vi "Cockpit_Demo.vi"() -> ()   [LabVIEW 2012]
uses:
  Sub_VIs/Instruments/SlipIndicator.ctl
  Sub_VIs/IMU_Functions/IMU_Data_Cluster.ctl
panel:
  in  "GPS/Baro_Vario":bool
  in  "GPS/Mag":bool
  in  "GPS/Baro_Alt":bool
  in  "ScaleUnit(F=m; T=feet)":bool
  out "AltitudeIndicator":picture
  out "VerticalSpeedIndicator":picture
  out "TurnBankPlaneIndicator":picture caption="Neue Grafik"
  in  "ScaleUnit(F=km/h; T=knots)":bool
  out "SpeedIndicator":picture
  out "TurnBankStdRate":bool
  out "AltitudeDigital":dbl
  out "VerticalSpeedDigital":dbl format="%.1f"
  out "HeadingDigital":dbl format="%.1f"
  out "Compass":picture
  in  "MultiWii Data Cluster":T1 {"Altitude abs [m]" format="%.2f"; "Baro T [°C]" format="%.1f"; "Baro P [mbara]" format="%.1f"; "GPS_coord[LON]" format="%#_9f"; "GPS_coord[LAT]" format="%#_9f"; "Altitude [m]" format="%.2f"}
  in  "SlipIndicator":dbl(knob) scale=-10.0..10.0
  out "GPS Data Valid?":bool
  out "GPS Sensor OK":bool
  out "UTC":string
  out "Local":string
  in  "Difference Local/UTC [h]":i32=1
  in  "Reset":bool
  in  "EXIT":bool
  in  "AH-Roll":dbl(knob) scale=-180.0..180.0
  in  "AH-Pitch":dbl(knob) scale=-90.0..90.0
  in  "Altitude":dbl(knob) scale=0.0..15000.0
  in  "Vert.Speed":dbl(knob) scale=-20.0..20.0
  in  "Kompass":dbl(knob) scale=0.0..360.0
  in  "Speed":dbl(knob) scale=0.0..200.0
  out "SlipIndicator":T2 scale=-10.0..10.0
  out "ArtificialHorizon":picture
  # "D - CF2811"
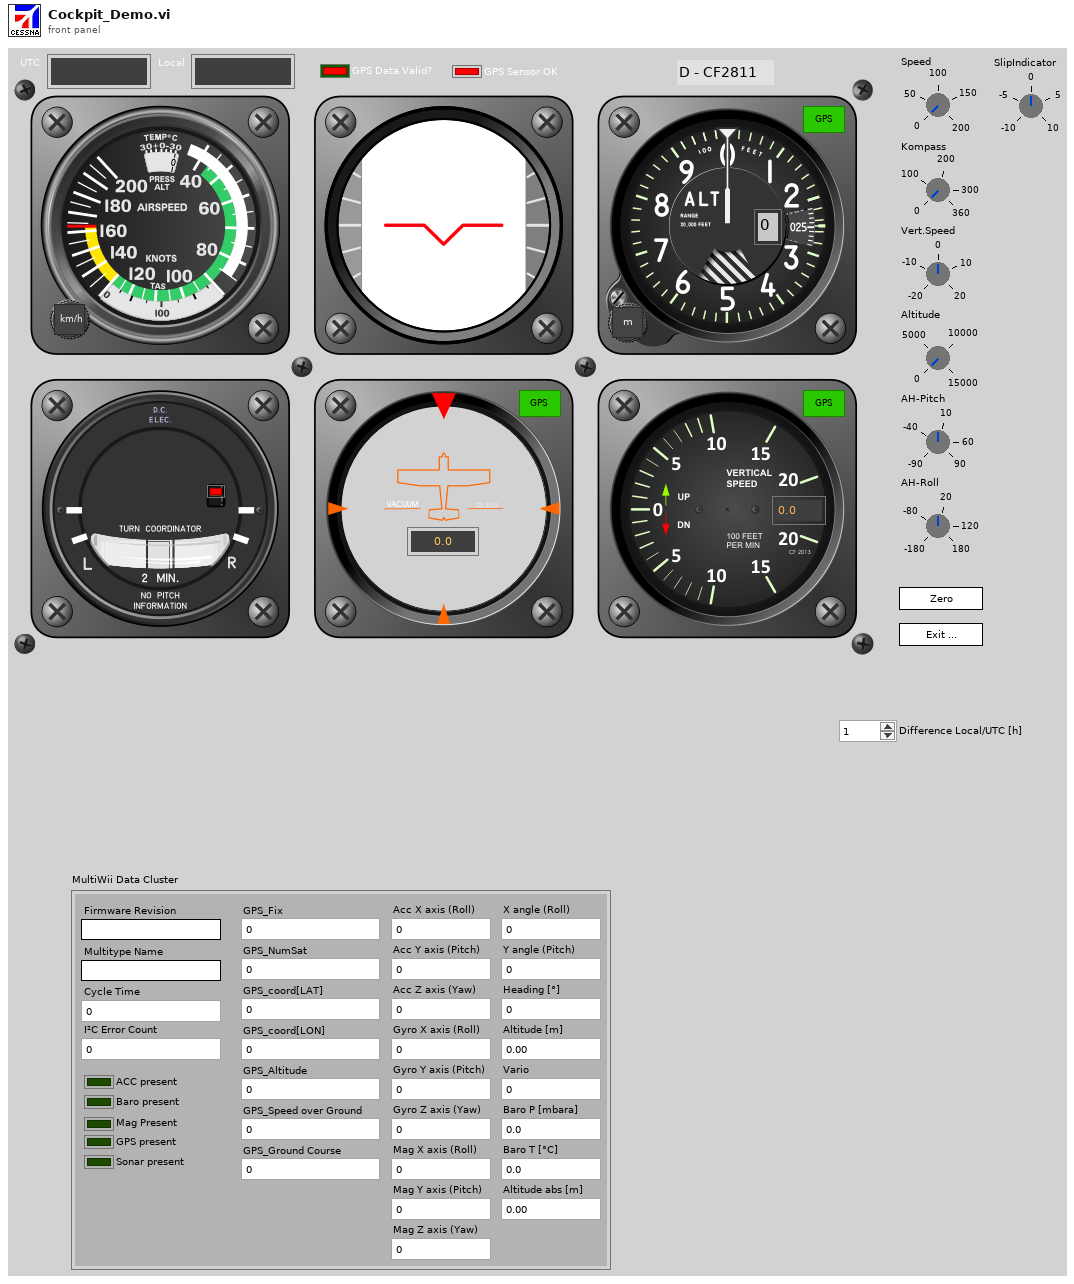
[diagram p1: front panel]
types:
  T1 = typedef "IMU_Data_Cluster.ctl" = cluster{"Firmware Revision":string, "Multitype Name":string, "Cycle Time":u16, "I²C Error Count":u16, "ACC present":bool, "Baro present":bool, "Mag Present":bool, "GPS present":bool, "Sonar present":bool, "Acc X axis (Roll)":dbl, "Acc Y axis (Pitch)":dbl, "Acc Z axis (Yaw)":dbl, "Gyro X axis (Roll)":dbl, "Gyro Y axis (Pitch)":dbl, "Gyro Z axis (Yaw)":dbl, "Mag X axis (Roll)":dbl, "Mag Y axis (Pitch)":dbl, "Mag Z axis (Yaw)":dbl, "X angle (Roll)":dbl, "Y angle (Pitch)":dbl, "Heading [°]":dbl, "Altitude [m]":dbl, "Vario":dbl, "GPS_Fix":u8, "GPS_NumSat":u8, "GPS_coord[LAT]":dbl, "GPS_coord[LON]":dbl, "GPS_Altitude":dbl, "GPS_Speed over Ground":dbl, "GPS_Ground Course":dbl, "Baro P [mbara]":dbl, "Baro T [°C]":dbl, "Altitude abs [m]":dbl}
  T2 = typedef "SlipIndicator.ctl" = dbl
  T3 = enum16{"GPS Altitude", "Baro absolute Altitude", "Baro Vario"}
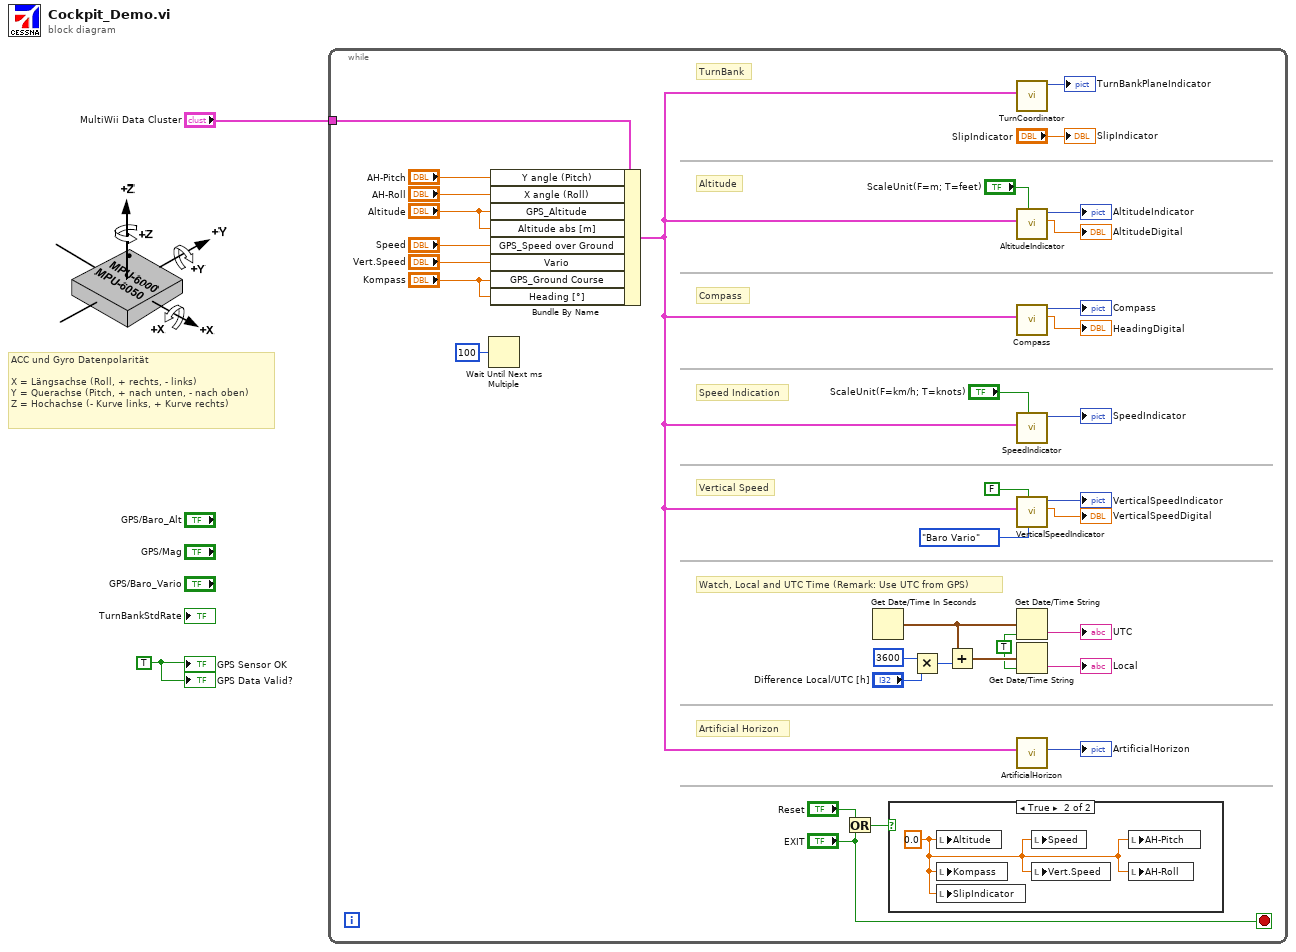
[diagram p0: block diagram]
diagram:
  w2 = TRUE
  # "ACC und Gyro Datenpolarität\n\nX = Längsachse (Roll, + rechts, - links)\nY = Querachse (Pitch, + nach unten, - nach oben)\nZ = Hochachse (- Kurve links, + Kurve rechts)"
  n1 = while {
    tunnel: "MultiWii Data Cluster" -> [w15]
    stop <- "EXIT" stop-if-true
    w28 = TRUE
    # "TurnBank"
    # "Watch, Local and UTC Time (Remark: Use UTC from GPS)"
    # "Artificial Horizon"
    # "Vertical Speed"
    # "Speed Indication"
    # "Compass"
    # "Altitude"
    n2 = Wait Until Next ms Multiple(millisecond multiple=u32 100 ("Vielfache von ms")) -> ()  [unwired: 1 out]
    n3 = Bundle By Name(cluster=w15, "Y angle (Pitch)"="AH-Pitch", "X angle (Roll)"="AH-Roll", "GPS_Altitude"="Altitude", "Altitude abs [m]"="Altitude", "GPS_Speed over Ground"="Speed", "Vario"="Vert.Speed", "GPS_Ground Course"="Kompass", "Heading [°]"="Kompass") -> (w3:T1)
    n4 = Or(x="Reset", y="EXIT") -> (x .or. y?=w35:bool)
    n5 = Get Date/Time In Seconds() -> (seconds since 1Jan1904=w30:timestamp)
    n6 = case shown="True" w35 {
      frame False {
      }
      frame True {
        w37 = 0.0 ("Altitude")
        n7 = local write "Altitude"(w37) -> ()
        n8 = local write "Kompass"(w37) -> ()
        n9 = local write "SlipIndicator"(w37) -> ()
        n10 = local write "Speed"(w37) -> ()
        n11 = local write "Vert.Speed"(w37) -> ()
        n12 = local write "AH-Pitch"(w37) -> ()
        n13 = local write "AH-Roll"(w37) -> ()
      }
    }
    n14 = Multiply(x=3600 ("number"), y="Difference Local/UTC [h]") -> (x*y=w27:i32)
    n15 = Add(x=w30, y=w27) -> (x+y=w29:timestamp)
    n16 = call "TurnCoordinator.vi"("MultiWii Data Cluster"=w3) -> ("TurnBankPlaneIndicator"=→"TurnBankPlaneIndicator":picture)  [unwired: 5 in, 5 out]
    n17 = call "AltitudeIndicator.vi"("GPS/Baro_Alt"="ScaleUnit(F=m; T=feet)", "MultiWii Data Cluster"=w3) -> ("Altitude  (/10000)"=→"AltitudeDigital":dbl, "AltitudeIndicator"=→"AltitudeIndicator":picture)  [unwired: 5 in, 3 out]
    n18 = call "Compass.vi"("MultiWii Data Cluster"=w3) -> ("Heading Digital"=→"HeadingDigital":dbl, "CompassGauge"=→"Compass":picture)  [unwired: 8 in, 1 out]
    n19 = call "SpeedIndicator.vi"("ScaleUnit(F=km/h; T=knots)"="ScaleUnit(F=km/h; T=knots)", "MultiWii Data Cluster"=w3) -> ("SpeedIndicator"=→"SpeedIndicator":picture)  [unwired: 8 in, 1 out]
    n20 = call "VerticalSpeedIndicator.vi"("SignalSource"=T3."Baro Vario", "ScaleUnit(F=m/s; T=Ft/min/100)"=FALSE, "MultiWii Data Cluster"=w3) -> ("VerticalSpeedDigital"=→"VerticalSpeedDigital":dbl, "VerticalSpeedIndicator"=→"VerticalSpeedIndicator":picture)  [unwired: 6 in, 1 out]
    n21 = Get Date/Time String(seconds (now)=w30, want seconds? (F)=w28) -> (time string=→"UTC":string)  [unwired: 1 in, 1 out]
    n22 = Get Date/Time String(seconds (now)=w29, want seconds? (F)=w28) -> (time string=→"Local":string)  [unwired: 1 in, 1 out]
    n23 = call "ArtificialHorizon.vi"("MultiWii Data Cluster"=w3) -> ("ArtificialHorizon"=→"ArtificialHorizon":picture)  [unwired: 9 in, 1 out]
    "SlipIndicator" <- "SlipIndicator"
  }
  "GPS Sensor OK" <- w2
  "GPS Data Valid?" <- w2
